vi "Отладка ВП (Главная).vi"() -> ()   [LabVIEW 2017]
doc: "This VI is part of Exercise 2-3 in the LabVIEW Basics I Course.\n\nFirst, fix the broken run arrow and then use the different debugging tools to see how they work."
panel:
  out "Результат":dbl format="%.2f"
  out "Случайное число":dbl format="%.2f"
  out "Произведение":dbl format="%.2f"
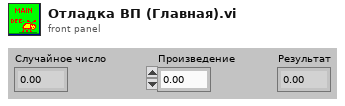
[diagram p1: front panel]
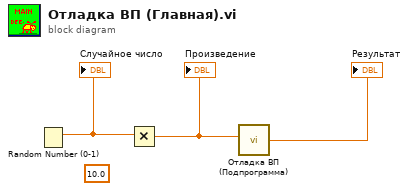
[diagram p0: block diagram]
diagram:
  (unwired) 10.0
  n1 = Random Number (0-1)() -> (number: 0 to 1=w2:dbl)
  "Случайное число" <- w2
  n2 = Multiply(x=w2) -> (x*y=w3:dbl)  [unwired: 1 in]
  "Произведение" <- w3
  n3 = call "Отладка ВП (Подпрограмма).vi"("Число"=w3) -> ("Результат"=→"Результат":dbl)
